vi "MGI Get Real Quadratic Roots SGL.vi"(9 "C":sgl, 10 "B":sgl, 11 "A":sgl) -> (2 "Root2":sgl, 3 "Root1":sgl)   [LabVIEW 2020]
doc: "Gets the real roots of the quadratic equation Ax^2 + Bx + C = 0. If there are no real roots, then both outputs are NaN. If there is a double root that is real, then both outputs are equal to the double root. If the coefficients correspond to a linear equation (i.e. A is zero) then Root1 is the solution to the linear equation and Root2 is NaN. This VI is configured to run as a subroutine.\n\nAuthored by Thomas Henage\nsupport@mooregoodideas.com\nwww.mooregoodideas.com\n\nCopyright (c) 2010, Moore Good Ideas, Inc.\n\nAll rights reserved.\n\nRedistribution and use in source and binary forms, with or without modification, are permitted provided that the following conditions are met:\n\n * Redistributions of source code must retain the above copyright notice, this list of conditions and the following disclaimer.\n * Redistributions in binary form must reproduce the above copyright notice, this list of conditions and the following disclaimer in the documentation and/or other materials provided with the distribution.\n * Neither the name of Moore Good Ideas, Inc. nor the names of its contributors may be used to endorse or promote products derived from this software without specific prior written permission.\n\nTHIS SOFTWARE IS PROVIDED BY THE COPYRIGHT HOLDERS AND CONTRIBUTORS \"AS IS\" AND ANY EXPRESS OR IMPLIED WARRANTIES, INCLUDING, BUT NOT LIMITED TO, THE IMPLIED WARRANTIES OF MERCHANTABILITY AND FITNESS FOR A PARTICULAR PURPOSE ARE DISCLAIMED. IN NO EVENT SHALL THE COPYRIGHT OWNER OR CONTRIBUTORS BE LIABLE FOR ANY DIRECT, INDIRECT, INCIDENTAL, SPECIAL, EXEMPLARY, OR CONSEQUENTIAL DAMAGES (INCLUDING, BUT NOT LIMITED TO, PROCUREMENT OF SUBSTITUTE GOODS OR SERVICES; LOSS OF USE, DATA, OR PROFITS; OR BUSINESS INTERRUPTION) HOWEVER CAUSED AND ON ANY THEORY OF LIABILITY, WHETHER IN CONTRACT, STRICT LIABILITY, OR TORT (INCLUDING NEGLIGENCE OR OTHERWISE) ARISING IN ANY WAY OUT OF THE USE OF THIS SOFTWARE, EVEN IF ADVISED OF THE POSSIBILITY OF SUCH DAMAGE."
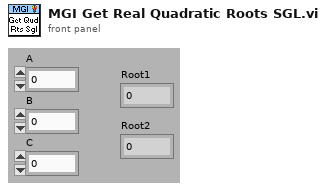
[diagram p1: front panel]
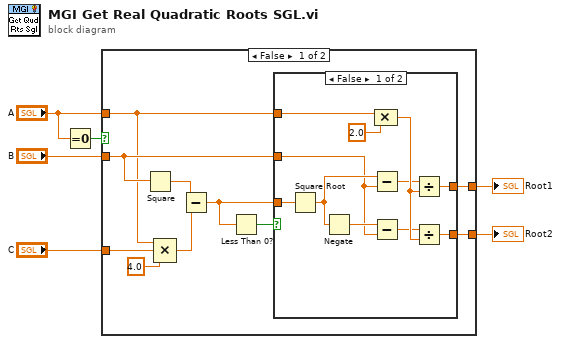
[diagram p0: block diagram]
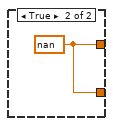
[diagram p2: hidden frame]
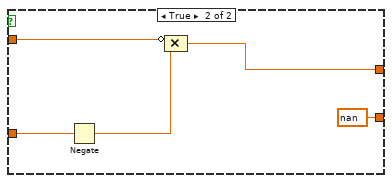
[diagram p3: hidden frame]
diagram:
  n1 = Equal To 0?(x="A") -> (x = 0?=w1:bool)
  n2 = case shown="False" w1 {
    tunnel: "C" -> [w16 w32]
    tunnel: "B" -> [w10 w31]
    tunnel: "A" -> [w9 _]
    tunnel: [w8 w29] -> w4
    tunnel: [w7 sgl nan] -> w3
    frame False {
      n3 = Square(x=w10) -> (x^2=w14:sgl)
      n4 = Compound Arithmetic op=MULTIPLY(w9, w16, sgl 4.0 ("value")) -> (w13:sgl)
      n5 = Subtract(x=w14, y=w13) -> (x-y=w11:sgl)
      n6 = Less Than 0?(x=w11) -> (x < 0?=w12:bool)
      n7 = case shown="False" w12 {
        tunnel: w11 -> [w27 _]
        tunnel: w10 -> [w24 _]
        tunnel: w9 -> [w23 _]
        tunnel: [w18 w28] -> w8
        tunnel: [w17 w28] -> w7
        frame False {
          n8 = Square Root(x=w27) -> (sqrt(x)=w26:sgl)
          n9 = Negate(x=w26) -> (-x=w25:sgl)
          n10 = Subtract(x=w26, y=w24) -> (x-y=w20:sgl)
          n11 = Subtract(x=w25, y=w24) -> (x-y=w19:sgl)
          n12 = Compound Arithmetic op=MULTIPLY(w23, sgl 2.0 ("value")) -> (w21:sgl)
          n13 = Divide(x=w20, y=w21) -> (x/y=w18:sgl)
          n14 = Divide(x=w19, y=w21) -> (x/y=w17:sgl)
        }
        frame True {
          w28 = sgl nan
        }
      }
    }
    frame True {
      n15 = Negate(x=w32) -> (-x=w30:sgl)
      n16 = Compound Arithmetic op=MULTIPLY(invert w31, w30) -> (w29:sgl)
    }
  }
  "Root2" <- w3
  "Root1" <- w4
